vi "Get Optimiser Strategy.vi"(8 "error in (no error)":errorcluster, 11 "Optimiser Cell in":refnum<class "Optimiser Cell.lvclass">) -> (0 "error out":errorcluster, 1 "Value":dbl, 2 "Optimisation Strategy":T1, 3 "Optimiser Cell out":refnum<class "Optimiser Cell.lvclass">)   [LabVIEW 2020, in "TALOS.lvlib" / "Run Utilities.lvlib" / "Optimiser Cell.lvclass"]
uses:
  Optimiser Cell.lvclass
  Optimisation Strategy.ctl
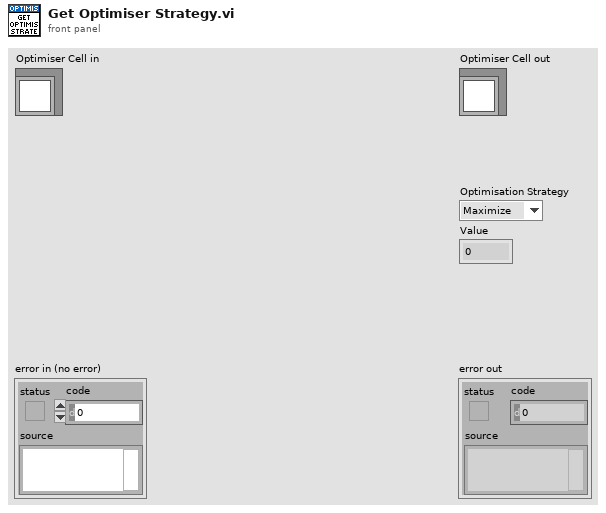
[diagram p1: front panel]
types:
  T1 = typedef "TALOS.lvlib/Run Utilities.lvlib/Optimiser Cell.lvclass/Optimisation Strategy.ctl" = enum16{"Maximize", "Minimize", "Value"}
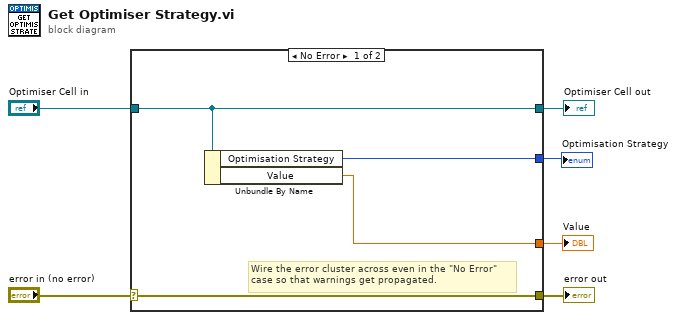
[diagram p0: block diagram]
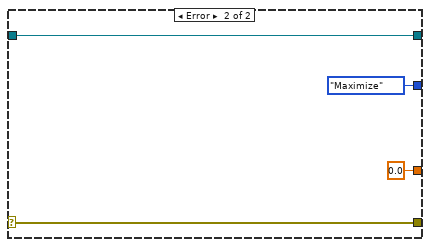
[diagram p2: hidden frame]
diagram:
  n1 = case shown="No Error" "error in (no error)" {
    selector: "error in (no error)" -> [w10 w14]
    tunnel: [w10 w14] -> w5
    tunnel: [w9 w13] -> w3
    tunnel: "Optimiser Cell in" -> [w9 w13]
    tunnel: [w8 Optimisation_Strategy."Maximize" ("Optimisation Strategy")] -> w2
    tunnel: [w7 0.0 ("Value")] -> w1
    frame No Error {
      # "Wire the error cluster across even in the \"No Error\"\ncase so that warnings get propagated."
      n2 = Unbundle By Name(w9) -> ("Optimisation Strategy"=w8:T1, "Value"=w7:dbl)
    }
    frame Error {
    }
  }
  "error out" <- w5
  "Optimiser Cell out" <- w3
  "Optimisation Strategy" <- w2
  "Value" <- w1
